vi "Run Bfr Rx - Postpend Null.vi"(8 "error in (no error)":errorcluster, 11 "Data Buffer in":u64 format="%016x") -> (0 "error out":errorcluster)   [LabVIEW 2019, in "UDP-Custom-Device Engine.lvlib"]
uses:
  UDP-Custom-Device Engine.lvlib
  <vilib>/NI VeriStand/VeriStand Data/Pointer Operations/Pointer.Write (I32).vi
  <vilib>/NI VeriStand/VeriStand Data/VeriStand Data.lvlib
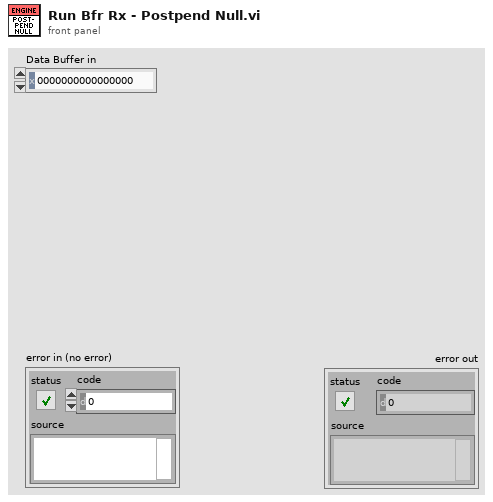
[diagram p1: front panel]
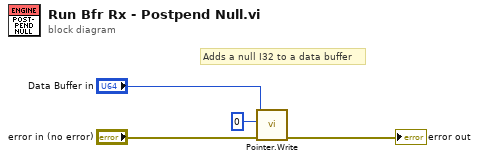
[diagram p0: block diagram]
diagram:
  # "Adds a null I32 to a data buffer"
  n1 = call-poly <vilib>:"Pointer.Write.vi"("error in (no error)"="error in (no error)", "value"=0, "pointer in"="Data Buffer in") -> ("error out"=→"error out":errorcluster)  [unwired: 6 in, 2 out]
